vi "Create.vi"(5 "private thread options":T1, 7 "public thread options":T1, 8 "error in (no error)":errorcluster, 10 "Public Threads":refnum<class "Thread.lvclass">[](array[class]), 11 "Private Threads":refnum<class "Thread.lvclass">[](array[class])) -> (0 "error out":errorcluster, 3 "Thread Manager":refnum<class "Thread Manager.lvclass">)   [LabVIEW 2019, in "DSF Core.lvlib" / "Thread Manager.lvclass"]
uses:
  Thread Manager.lvclass
  Thread/Thread.lvclass
  Thread/Thread Options.ctl
  <vilib>/NI/Memory Manager/Classes/Pointer/Pointer.lvclass/Pointer.ctl
  Pointers/Error/Error Pointer.lvclass/Error Pointer.ctl
  Thread/Thread.lvclass/Thread.ctl
  Thread Manager.lvclass/Thread Manager.ctl
  <vilib>/NI/Memory Manager/Classes/Pointer/Is Null.vi
  <vilib>/NI/Memory Manager/Classes/Pointer/Deallocate.vi
  <vilib>/NI/Memory Manager/Classes/Pointer/Get Address.vi
  <vilib>/NI/Memory Manager/Classes/Pointer/Encapsulate.vi
  <vilib>/NI/Memory Manager/Classes/Pointer/Check Null Pointer.vi
  <vilib>/NI/Memory Manager/Classes/Pointer/Check Length.vi
  <vilib>/NI/Memory Manager/Classes/Pointer/Set Address.vi
  <vilib>/NI/Memory Manager/Classes/Pointer/Set Size.vi
  <vilib>/NI/Memory Manager/Classes/Pointer/Set Internal.vi
  Pointers/Error/Write Error Pointer.vi
  Pointers/Error/Error Size.vi
  <vilib>/NI/Memory Manager/Classes/Pointer/Get Internal.vi
  <vilib>/NI/Memory Manager/Classes/Pointer/Errors.vi
  <vilib>/NI/Memory Manager/Classes/Pointer/Zone.vi
  <vilib>/NI/Memory Manager/Classes/Pointer/Null Pointer.vi
  <vilib>/NI/Memory Manager/Classes/Pointer/Get Size.vi
  <vilib>/NI/Memory Manager/Classes/Pointer/Check Bounds (Pointer).vi
  <vilib>/NI/Memory Manager/Classes/Pointer/Write.vi
  <vilib>/NI/Memory Manager/Classes/Pointer/Write 1D U8.vi
  <vilib>/NI/Memory Manager/Classes/Pointer/Clear.vi
  <vilib>/NI/Memory Manager/Classes/Pointer/Create Error.vi
  <vilib>/NI/Memory Manager/Classes/Pointer/Out of Bounds.vi
  <vilib>/NI/Memory Manager/Classes/Pointer/Write (No Check).vi
  <vilib>/NI/Memory Manager/Classes/Pointer/Write (No Check) 1D U8.vi
  <vilib>/NI/Memory Manager/Classes/Pointer/Check Move.vi
  <vilib>/NI/Memory Manager/Classes/Pointer/Clear (No Check).vi
  <vilib>/NI/Memory Manager/VIs/New Error Cluster.vi
  <vilib>/NI/Memory Manager/VIs/New Error Cluster (512B).vi
  <vilib>/NI/Memory Manager/VIs/Set Error Status.vi
  <vilib>/NI/Memory Manager/VIs/Set Error Code.vi
  <vilib>/NI/Memory Manager/VIs/Set Error Source.vi
  <vilib>/NI/Memory Manager/Constants/Constants.vi
  <vilib>/NI/Memory Manager/Constants/Library Name.vi
  <vilib>/NI/Memory Manager/Classes/Pointer/Pointer Error Info.vi
  <vilib>/NI/Memory Manager/VIs/Write String to Source.vi
  <vilib>/NI/Memory Manager/Constants/Pointer Class Name.vi
  <vilib>/NI/Memory Manager/Classes/Pointer/Write Pointer Size to Error.vi
  <vilib>/NI/Memory Manager/VIs/Write Numeric to Source.vi
  <vilib>/NI/Memory Manager/VIs/Write Numeric Scalar to Source (Base10 U64).vi
  <vilib>/NI/Memory Manager/Classes/Pointer/Check Count.vi
  <vilib>/NI/Memory Manager/Classes/Pointer/Check Bounds (Power of 2).vi
  <vilib>/NI/Memory Manager/Classes/Pointer/Check Bounds.vi
  <vilib>/NI/Memory Manager/Classes/Pointer/Check Bounds (Buffer).vi
  <vilib>/NI/Memory Manager/Classes/Pointer/Buffer Underflow.vi
  Pointers/Error/Error Pointer.lvclass
  C:/Program Files (x86)/National Instruments/LabVIEW 2019/vi.lib/NI/Memory Manager/Classes/Pointer/Pointer.lvclass
  <vilib>/NI/Memory Manager/Classes/Pointer/Pointer.lvclass
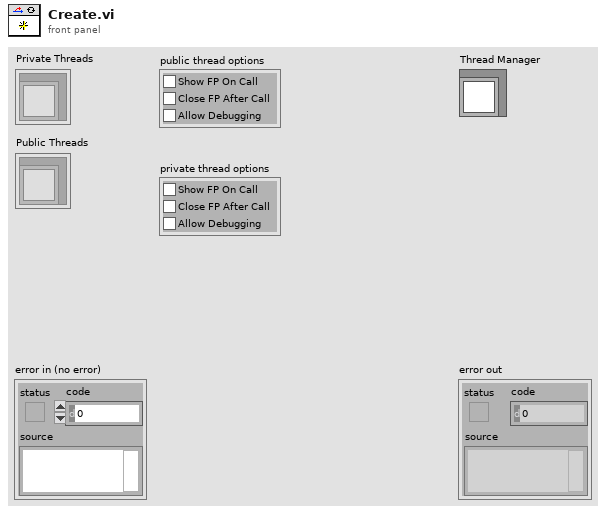
[diagram p1: front panel]
types:
  T1 = typedef "DSF Core.lvlib/Thread.lvclass/Thread Options.ctl" = cluster{"Show FP On Call":bool, "Close FP After Call":bool, "Allow Debugging":bool}
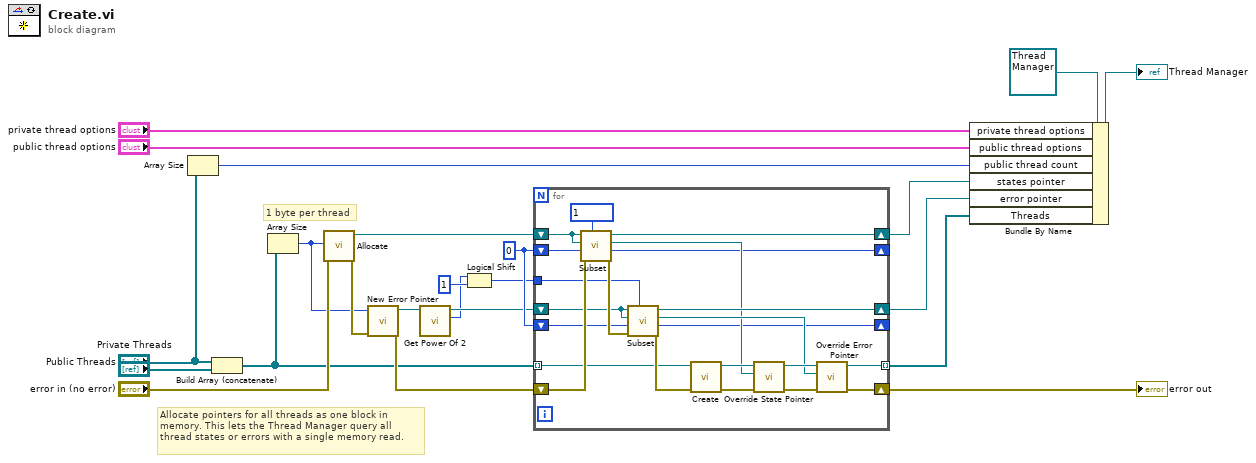
[diagram p0: block diagram]
diagram:
  w7 = u64 0 ("offset (0)")
  # "Allocate pointers for all threads as one block in memory. This lets the Thread Manager query all thread states or errors with a single memory read."
  # "1 byte per thread"
  n1 = Array Size(array="Public Threads") -> (size(s)=w16:i32)
  n2 = Build Array (concatenate)("Public Threads", "Private Threads") -> (w1:refnum<class "Thread.lvclass">[])
  n3 = Array Size(array=w1) -> (size(s)=w12:i32)
  n4 = call <vilib>:"Allocate.vi"("error in (no error)"="error in (no error)", "size"=w12) -> ("error out"=w14:errorcluster, "Pointer out"=w19:refnum<class "Pointer.lvclass">)  [unwired: 8 in]
  n5 = call "New Error Pointer.vi"("error in (no error)"=w14, "count (1)"=w12) -> ("error out"=w13:errorcluster, "Error Pointer"=w9:refnum<class "Error Pointer.lvclass">)  [unwired: 8 in]
  n6 = call "Get Power Of 2.vi"("Error Pointer in"=w9) -> ("power of 2"=w5:i16, "Error Pointer out"=w6:refnum<class "Error Pointer.lvclass">)  [unwired: 9 in]
  n7 = Logical Shift(y=w5, x=i64 1) -> (x << y=w4:i64)
  n8 = for {
    tunnel: w1 -> [w33] mode=indexing
    shift-right: [w37] -> w17
    shift-left: w13 -> [w36]
    shift-right: [w42] -> w15
    shift-left: w19 -> [w40]
    shift-right: [w25] -> _
    shift-left: w7 -> [w41]
    shift-right: [w32] -> w11
    shift-left: w6 -> [w31]
    shift-right: [w24] -> _
    shift-left: w7 -> [w30]
    tunnel: [w29] -> w10 mode=indexing
    tunnel: w4 -> [w28]
    n9 = call <vilib>:"Subset.vi"("length (-1: rest)"=i64 1, "error in (no error)"=w36, "offset (0)"=w41, "subset Pointer type"=w40, "base Pointer in"=w40) -> ("error out"=w35:errorcluster, "offset + size"=w25:u64, "subset Pointer"=w26:refnum<class "Pointer.lvclass">, "base Pointer out"=w42:refnum<class "Pointer.lvclass">)  [unwired: 3 in]
    n10 = call <vilib>:"Subset.vi"("length (-1: rest)"=w28, "error in (no error)"=w35, "offset (0)"=w30, "subset Pointer type"=w31, "base Pointer in"=w31) -> ("error out"=w34:errorcluster, "offset + size"=w24:u64, "subset Pointer"=w27:refnum<class "Error Pointer.lvclass">, "base Pointer out"=w32:refnum<class "Error Pointer.lvclass">)  [unwired: 3 in]
    n11 = call-dynamic "Create.vi"("error in (no error)"=w34, "Thread in"=w33) -> ("error out"=w43:errorcluster, "Thread out"=w45:refnum<class "Thread.lvclass">)  [unwired: 8 in]
    n12 = call "Override State Pointer.vi"("error in (no error)"=w43, "new state pointer"=w26, "Thread in"=w45) -> ("error out"=w39:errorcluster, "Thread out"=w38:refnum<class "Thread.lvclass">)  [unwired: 7 in]
    n13 = call "Override Error Pointer.vi"("error in (no error)"=w39, "new error pointer"=w27, "Thread in"=w38) -> ("error out"=w37:errorcluster, "Thread out"=w29:refnum<class "Thread.lvclass">)  [unwired: 7 in]
  }
  "error out" <- w17
  n14 = Bundle By Name(cluster=refnum<class "Thread Manager.lvclass"> refnum ("Thread Manager in"), "private thread options"="private thread options", "public thread options"="public thread options", "public thread count"=w16, "states pointer"=w15, "error pointer"=w11, "Threads"=w10) -> (→"Thread Manager":refnum<class "Thread Manager.lvclass">)
